vi "Update Attributes Actors.vi"(7 "Attributes in":refnum<class "Attributes.lvclass">, 10 "Actors":refnum<class "Actor.lvclass">[](array[class])) -> (5 "Attributes out":refnum<class "Attributes.lvclass">)   [LabVIEW 2020, in "jettl.lvlib"]
uses:
  jettl.lvlib
  Attributes/Attributes.lvclass
  Attributes Metadata/Attributes Metadata.lvclass
  Transport/Transport.lvclass
  Msg/Msg.lvclass
  Msgs.ctl
  Actor/Actor.lvclass
  Attributes.ctl
  Base Attributes/Base Attributes.lvlib
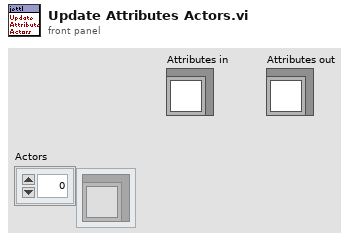
[diagram p1: front panel]
types:
  T1 = typedef "jettl.lvlib/Attributes.ctl" = cluster{"Attributes Metadata":refnum<class "Attributes Metadata.lvclass">, "Unified Msgs":T2, "Unified Leaf":bool, "Edge Actors":refnum<class "Actor.lvclass">[], "Core Actors":refnum<class "Actor.lvclass">[], "Parent Attributes":refnum<class "Attributes.lvclass">, "Root":bool, "Alias":string, "UID":i32, "Transport":refnum<class "Transport.lvclass">, "VI Ref":refnum<vi>, "Actors":refnum<class "Actor.lvclass">[]}
  T2 = typedef "jettl.lvlib/Msgs.ctl" = set{refnum<class "Msg.lvclass">}
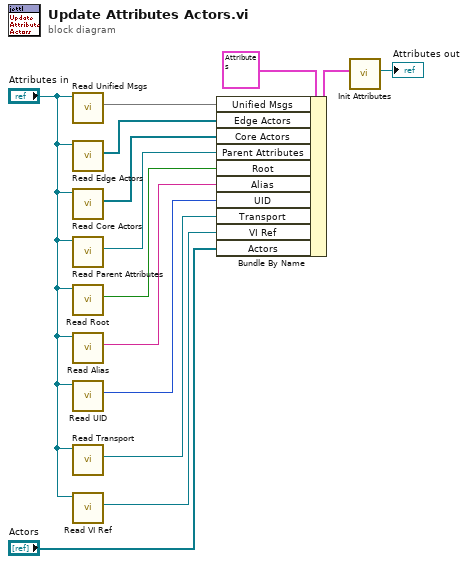
[diagram p0: block diagram]
diagram:
  n1 = call-dynamic "Read Unified Msgs.vi"("Attributes in"="Attributes in") -> ("Unified Msgs"=w5:T2)  [unwired: 10 in]
  n2 = call-dynamic "Read Edge Actors.vi"("Attributes in"="Attributes in") -> ("Edge Actors"=w4:refnum<class "Actor.lvclass">[])  [unwired: 10 in]
  n3 = call-dynamic "Read Core Actors.vi"("Attributes in"="Attributes in") -> ("Core Actors"=w6:refnum<class "Actor.lvclass">[])  [unwired: 10 in]
  n4 = call-dynamic "Read Parent Attributes.vi"("Attributes in"="Attributes in") -> ("Parent Attributes"=w7:refnum<class "Attributes.lvclass">)  [unwired: 10 in]
  n5 = call-dynamic "Read Root.vi"("Attributes in"="Attributes in") -> ("Root"=w8:bool)  [unwired: 10 in]
  n6 = call-dynamic "Read Alias.vi"("Attributes in"="Attributes in") -> ("Alias"=w9:string)  [unwired: 10 in]
  n7 = call-dynamic "Read UID.vi"("Attributes in"="Attributes in") -> ("UID"=w1:i32)  [unwired: 10 in]
  n8 = call-dynamic "Read Transport.vi"("Attributes in"="Attributes in") -> ("Transport"=w2:refnum<class "Transport.lvclass">)  [unwired: 10 in]
  n9 = call-dynamic "Read VI Ref.vi"("Attributes in"="Attributes in") -> ("VI Ref"=w10:refnum<vi>)  [unwired: 10 in]
  n10 = Bundle By Name(cluster=T1 {"Attributes Metadata"=refnum, "Unified Msgs"={}, "Unified Leaf"=FALSE, "Edge Actors"=[], "Core Actors"=[], "Parent Attributes"=refnum, "Root"=FALSE, "Alias"="", "UID"=0, "Transport"=refnum, "VI Ref"=refnum, "Actors"=[]} ("Attributes"), "Unified Msgs"=w5, "Edge Actors"=w4, "Core Actors"=w6, "Parent Attributes"=w7, "Root"=w8, "Alias"=w9, "UID"=w1, "Transport"=w2, "VI Ref"=w10, "Actors"="Actors") -> (w12:T1)
  n11 = call "Init Attributes.vi"("Attributes"=w12) -> ("Attributes"=→"Attributes out":refnum<class "Attributes.lvclass">)  [unwired: 10 in]
